vi "test Non Match Fails The Test.vi"(8 "error in (no error)":errorcluster, 11 "TestCase in":refnum<class "String Regex Test Case.lvclass">) -> (0 "error out":errorcluster, 3 "TestCase out":refnum<class "String Regex Test Case.lvclass">)   [LabVIEW 2015, in "String Regex Test Case.lvclass"]
uses:
  String Regex Test Case.lvclass
  <vilib>/addons/_JKI Toolkits/VI Tester/TestCase.llb/TestCase.lvclass
  VITAC.lvlib
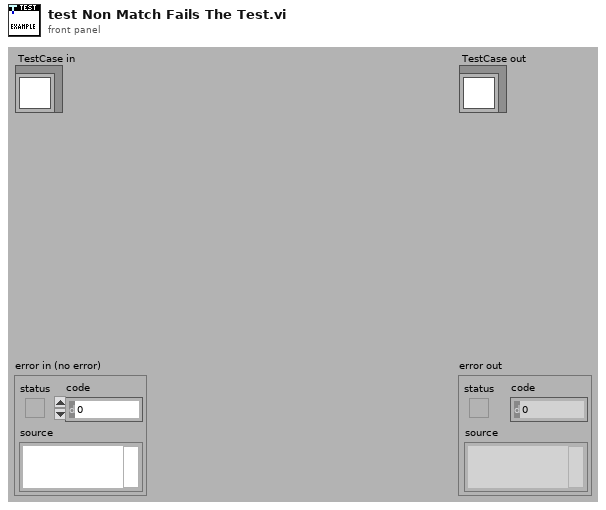
[diagram p1: front panel]
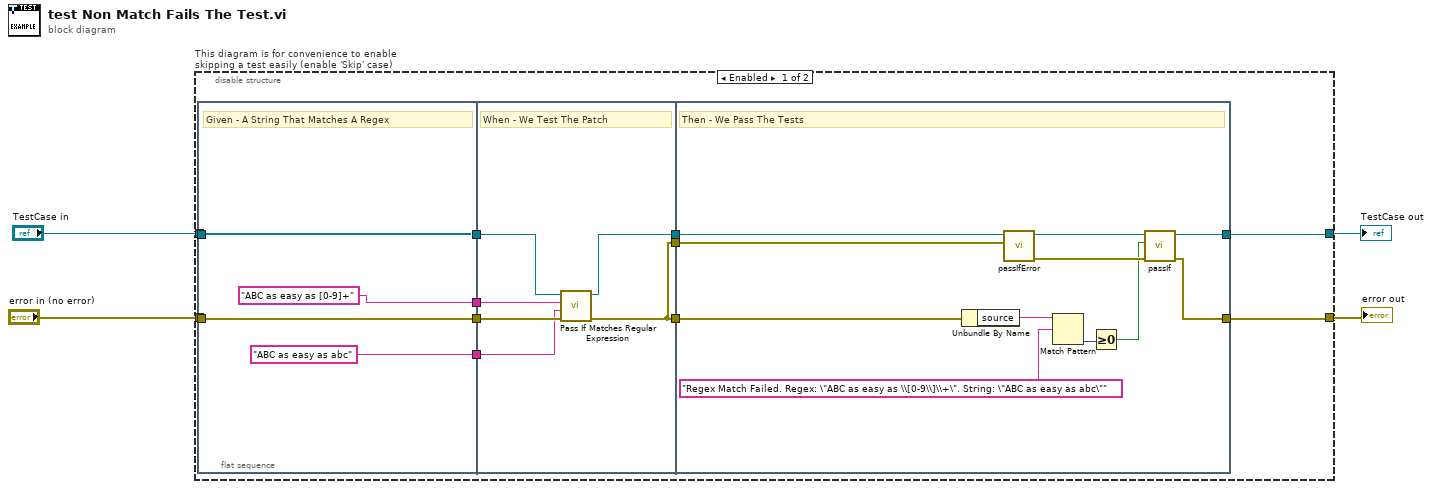
[diagram p0: block diagram]
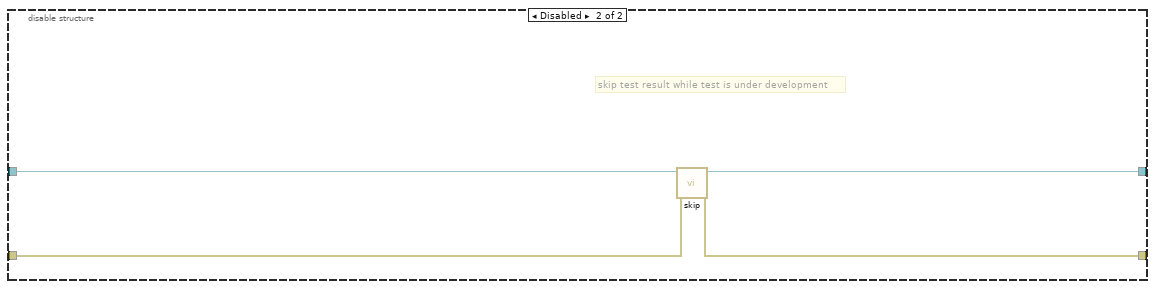
[diagram p2: hidden frame]
diagram:
  n1 = disable-structure "This diagram is for convenience to enable skipping a test easily (enable 'Skip' case)" shown="Enabled" {
    disable-tunnel: "TestCase in" -> [w12 w40]
    disable-tunnel: [w10 w38] -> w1
    disable-tunnel: [w9 w39] -> w3
    disable-tunnel: "error in (no error)" -> [w11 w37]
    frame Enabled {
      n2 = flat-sequence {
        tunnel: w11 -> [w18]
        tunnel: w12 -> [w19]
        tunnel: [w19] -> w15
        tunnel: [w18] -> w14
        tunnel: ["ABC as easy as abc" ("actual")] -> w8
        tunnel: ["ABC as easy as [0-9]+" ("actual")] -> w7
        tunnel: [w23] -> w13
        tunnel: w15 -> [w24]
        tunnel: w14 -> [w25]
        tunnel: w8 -> [w22]
        tunnel: w7 -> [w21]
        tunnel: [w20] -> w6
        tunnel: [w20] -> w5
        tunnel: w13 -> [w36]
        tunnel: [w30] -> w10
        tunnel: [w27] -> w9
        tunnel: w6 -> [w34]
        tunnel: w5 -> [w33]
        frame #0 {
          # "Given - A String That Matches A Regex"
        }
        frame #1 {
          # "When - We Test The Patch"
          n3 = call "Pass If Matches Regular Expression.vi"("error in (no error)"=w25, "actual"=w22, "regular expression"=w21, "TestCase in"=w24) -> ("error out"=w20:errorcluster, "TestCase out"=w23:refnum<class "String Regex Test Case.lvclass">)  [unwired: 6 in]
        }
        frame #2 {
          # "Then - We Pass The Tests"
          n4 = Unbundle By Name(w33) -> ("source"=w32:string)
          n5 = call-dynamic "passIfError.vi"("error"=w34, "TestCase in"=w36) -> ("error out"=w29:errorcluster, "TestCase out"=w35:refnum<class "String Regex Test Case.lvclass">)  [unwired: 8 in]
          n6 = Match Pattern(string=w32, regular expression="Regex Match Failed. Regex: \"ABC as easy as \\[0-9\\]\\+\". String: \"ABC as easy as abc\"" ("actual")) -> (offset past match=w31:i32)  [unwired: 1 in, 3 out]
          n7 = Greater Or Equal To 0?(x=w31) -> (x >= 0?=w28:bool)
          n8 = call-dynamic "passIf.vi"("error in (no error)"=w29, "pass"=w28, "TestCase in"=w35) -> ("error out"=w27:errorcluster, "TestCase out"=w30:refnum<class "String Regex Test Case.lvclass">)  [unwired: 7 in]
        }
      }
    }
    frame Disabled {
      # "skip test result while test is under development"
      n9 = call <vilib>:"skip.vi"("error in (no error)"=w37, "TestCase in"=w40) -> ("error out"=w39:errorcluster, "TestCase out"=w38:refnum<class "String Regex Test Case.lvclass">)  [unwired: 8 in]
    }
  }
  "error out" <- w3
  "TestCase out" <- w1
